vi "10 Rings, Strings, and Tables.vi"() -> ()   [LabVIEW 2020]
uses:
  _Subs/OpenDiagram/Open_XControl.xctl
panel:
  in  "OpenDiag":refnum<vi>(xcontrol)
  out "where is the fox?":string
  out "more text":string
  in  "Listbox":i32(listbox)=2
  out "Table Indicator":string[][](table)
  out "Labels":string
  in  "Enum":enum16{"Tall", "Medium", "Short"}(ring)=enum."Medium"
  in  "Ring":u16(ring)=2 items=["Tall", "Medium", "Short"]
  # "10 Rings, Strings, and Tables\nThis code shows different ways of using tables, strings, and rings\n\nInstructions:\n1. Hit the Run arrow and see what happens.\n2. Try selecting a different value in the ring or list box and run again"
  # "Right Btn click and Edit Items..."
  # "Hit Cmd E to see the diagram (code)"
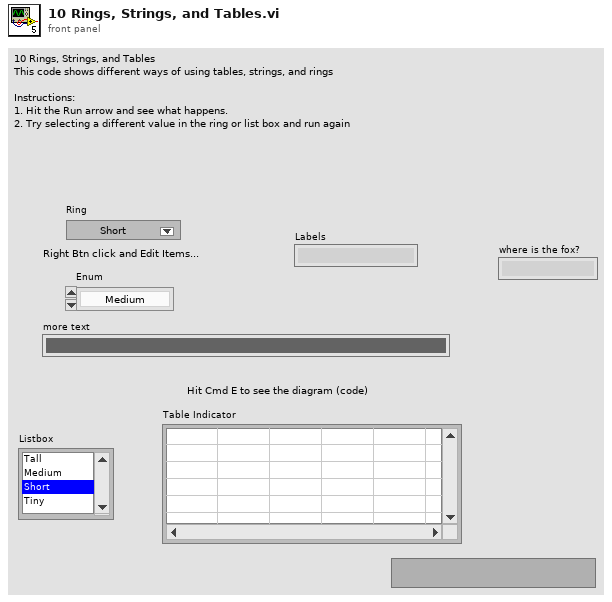
[diagram p1: front panel]
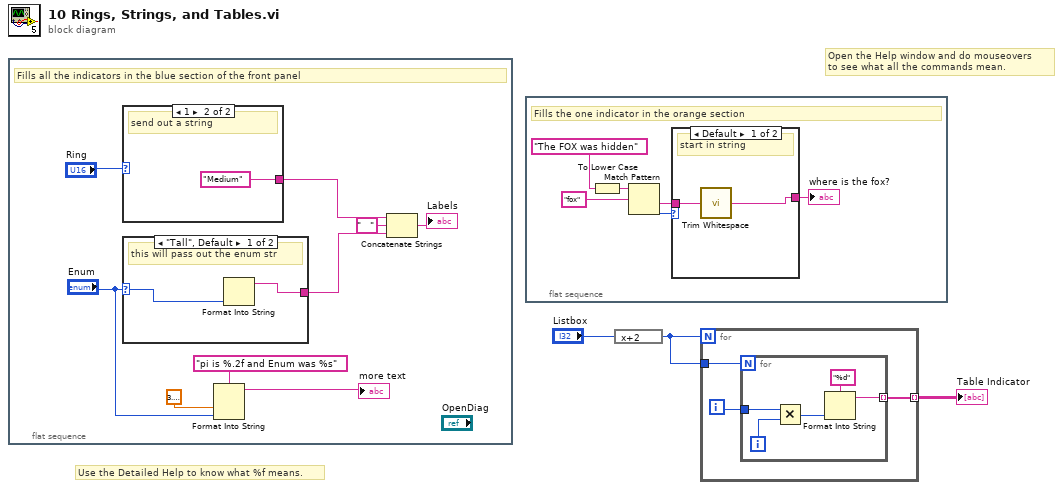
[diagram p0: block diagram]
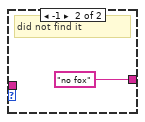
[diagram p2: hidden frame]
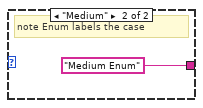
[diagram p3: hidden frame]
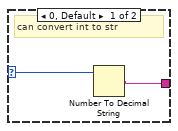
[diagram p4: hidden frame]
diagram:
  # "Use the Detailed Help to know what %f means."
  # "Open the Help window and do mouseovers\nto see what all the commands mean."
  n1 = flat-sequence {
    frame #0 {
      # "Fills all the indicators in the blue section of the front panel"
      n2 = case shown="1" "Ring" {
        selector: "Ring" -> [w17 _]
        tunnel: [w16 "Medium"] -> w10
        frame 0, Default {
          # "can convert int to str"
          n3 = Number To Decimal String(number=w17) -> (decimal integer string=w16:string)  [unwired: 1 in]
        }
        frame 1 {
          # "send out a string"
        }
      }
      n4 = case shown="\"Tall\", Default" "Enum" {
        selector: "Enum" -> [w14 _]
        tunnel: [w13 "Medium Enum"] -> w11
        frame "Tall", Default {
          # "this will pass out the enum str"
          n5 = Format Into String(w14) -> (resulting string=w13:string)  [unwired: 3 in, 1 out]
        }
        frame "Medium" {
          # "note Enum labels the case"
        }
      }
      n6 = Format Into String(format string="pi is %.2f and Enum was %s", 3.141592653589793, "Enum") -> (resulting string=→"more text":string)  [unwired: 2 in, 1 out]
      n7 = Concatenate Strings(w10, "   " ("string"), w11) -> (→"Labels":string)
    }
  }
  n8 = flat-sequence {
    frame #0 {
      # "Fills the one indicator in the orange section"
      n9 = To Lower Case(string="The FOX was hidden" ("format string")) -> (all lower case string=w22:string)
      n10 = Match Pattern(string=w22, regular expression="fox") -> (after substring=w19:string, offset past match=w21:i32)  [unwired: 1 in, 2 out]
      n11 = case shown="Default" w21 {
        tunnel: [w25 "no fox" ("regular expression")] -> w20
        tunnel: w19 -> [w26 _]
        frame Default {
          # "start in string"
          n12 = call <vilib>:"Trim Whitespace.vi"("string"=w26) -> ("trimmed string"=w25:string)  [unwired: 1 in]
        }
        frame -1 {
          # "did not find it"
        }
      }
      "where is the fox?" <- w20
    }
  }
  n13 = expression code="x+2"("Listbox") -> (w2:i32)
  n14 = for {
    N: w2 -> [_]
    tunnel: w2 -> [w30]
    tunnel: [w29] -> w3 mode=indexing
    i -> [w28]
    n15 = for {
      N: w30 -> [_]
      tunnel: [w34] -> w29 mode=indexing
      tunnel: w28 -> [w33]
      i -> [w32]
      n16 = Multiply(x=w33, y=w32) -> (x*y=w31:i32)
      n17 = Format Into String(format string="%d", w31) -> (resulting string=w34:string)  [unwired: 2 in, 1 out]
    }
  }
  "Table Indicator" <- w3
